vi "sub vi - send mail with attach v4.vi"(0 "TO:":string, 1 "subject":string, 5 "from":string, 7 "out going server":string, 9 "message":string, 11 "username":string, 12 "password":string, 13 "Attachements":path[](array[path])) -> (15 "error out":errorcluster)   [LabVIEW 2013]
uses:
  <vilib>/smtpClient/Set Message Text.vi
  <vilib>/smtpClient/LabVIEWSMTPClient.lvlib
panel:
  in  "Tab Control":enum32{"Page 1", "Page 2"}(tab)
  in  "Mail To:":string[](array[string])
  # "SENDING MAIL"
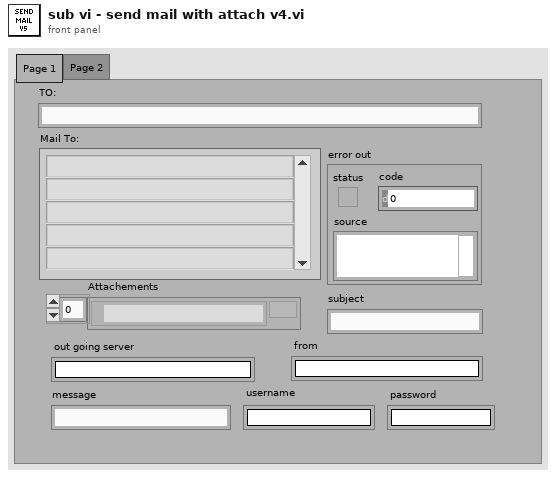
[diagram p1: front panel]
types:
  T1 = typedef "LabVIEWSMTPClient.lvlib/SmtpClientHandle.ctl" = refnum<k1>
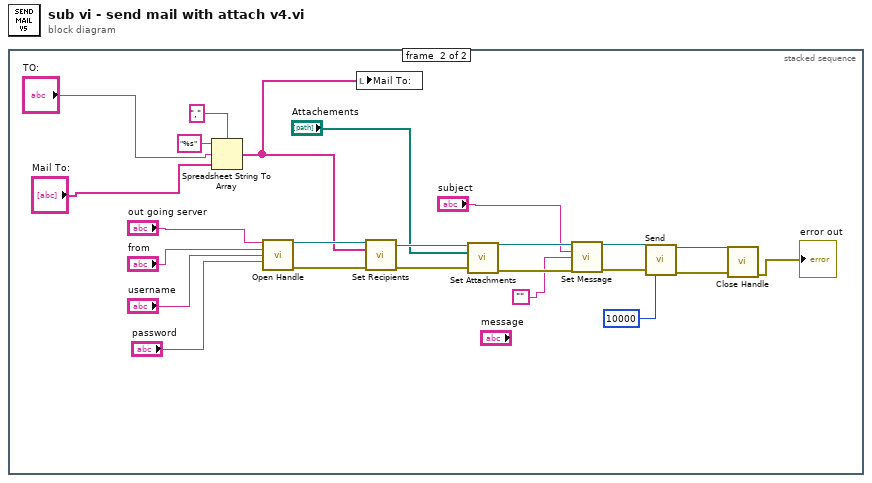
[diagram p0: block diagram]
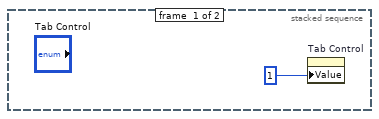
[diagram p2: hidden frame]
diagram:
  n1 = stacked-sequence {
    frame #0 {
      n2 = property on="Tab Control" class="TabCtl (strict)"("Value"=1) -> ()  [unwired: 2 in, 2 out]
    }
    frame #1 {
      n3 = Spreadsheet String To Array(delimiter (Tab)=",", format string="%s", spreadsheet string="TO:", array type (2D Dbl)="Mail To:") -> (array=w4:string[])
      n4 = call <vilib>:"Open Handle.vi"("server address"="out going server", "from"="from", "username"="username", "password"="password") -> ("handle out"=w21:T1, "error out"=w20:errorcluster)  [unwired: 10 in]
      n5 = local write "Mail To:"(w4) -> ()
      n6 = call <vilib>:"Set Recipients.vi"("handle in"=w21, "to"=w4, "error in (no error)"=w20) -> ("handle out"=w19:T1, "error out"=w16:errorcluster)  [unwired: 11 in]
      n7 = call <vilib>:"Set Attachments.vi"("handle in"=w19, "attachments"="Attachements", "error in (no error)"=w16) -> ("handle out"=w18:T1, "error out"=w15:errorcluster)  [unwired: 11 in]
      n8 = call-poly <vilib>:"Set Message.vi"("handle in"=w18, "subject"="subject", "plain text message"="", "error in (no error)"=w15) -> ("handle out"=w17:T1, "error out"=w14:errorcluster)  [unwired: 10 in]
      n9 = call <vilib>:"Send.vi"("handle in"=w17, "error in (no error)"=w14, "timeout in ms (10000)"=10000) -> ("handle out"=w13:T1, "error out"=w12:errorcluster)  [unwired: 10 in, 1 out]
      n10 = call <vilib>:"Close Handle.vi"("handle in"=w13, "error in (no error)"=w12) -> ("error out"=→"error out":errorcluster)  [unwired: 12 in, 1 out]
    }
  }
